vi "Get GUID Controls on Constants VI.vi"(8 "error in":errorcluster, 11 "VI in":refnum<vi>) -> (0 "error out":errorcluster, 2 "GUID controls":refnum<vi>[](array[refnum]), 3 "VI out":refnum<vi>)   [LabVIEW 2020, in "Utility.lvlib"]
uses:
  Utility.lvlib
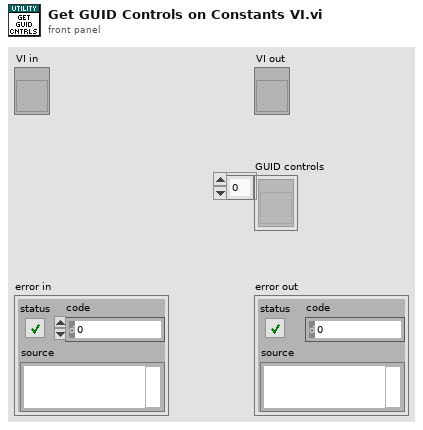
[diagram p1: front panel]
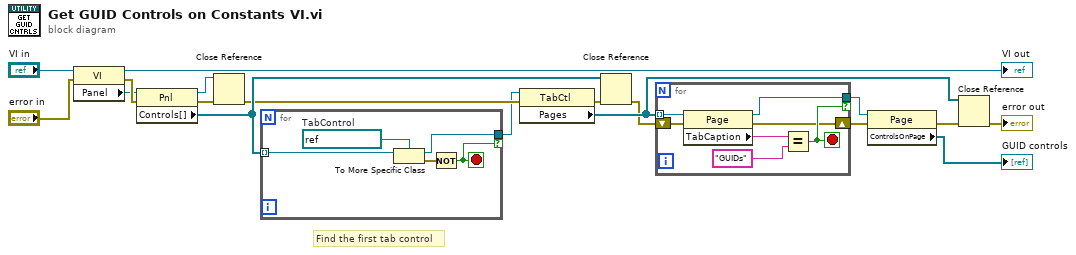
[diagram p0: block diagram]
diagram:
  # "Find the first tab control"
  n1 = property class="VI"(reference="VI in", error in="error in") -> (reference out=→"VI out":refnum<vi>, error out=w7:errorcluster, "Panel"=w3:refnum<vi>)
  n2 = property class="Pnl"(reference=w3, error in=w7) -> (reference out=w9:refnum<vi>, error out=w8:errorcluster, "Controls[]"=w15:refnum<vi>[])
  n3 = Close Reference(reference=w9, error in (no error)=w8) -> (error out=w10:errorcluster)
  n4 = for {
    tunnel: w15 -> [w23] mode=indexing
    tunnel: [w21] -> w2 if=w19
    stop <- w19 stop-if-true
    w22 = refnum<vi> refnum  # TabControl
    n5 = To More Specific Class(target class=w22, reference=w23) -> (specific class reference=w21:refnum<vi>, error out=w20:errorcluster)  [unwired: 1 in]
    n6 = Not(x=w20) -> (.not. x?=w19:bool)
  }
  n7 = property class="TabCtl"(reference=w2, error in=w10) -> (error out=w11:errorcluster, "Pages"=w17:refnum<vi>[])  [unwired: 1 out]
  n8 = Close Reference(reference=w15, error in (no error)=w11) -> (error out=w14:errorcluster)
  n9 = for {
    tunnel: w17 -> [w30] mode=indexing
    tunnel: [w29] -> w1 if=w28
    shift-right: [w26] -> w12
    shift-left: w14 -> [w27]
    stop <- w28 stop-if-true
    n10 = property class="Page"(reference=w30, error in=w27) -> (reference out=w29:refnum<vi>, error out=w26:errorcluster, "TabCaption"=w24:string)
    n11 = Equal?(x=w24, y="GUIDs") -> (x = y?=w28:bool)
  }
  n12 = property class="Page"(reference=w1, error in=w12) -> (error out=w13:errorcluster, "ControlsOnPage"=→"GUID controls":refnum<vi>[])  [unwired: 1 out]
  n13 = Close Reference(reference=w17, error in (no error)=w13) -> (error out=→"error out":errorcluster)
